vi "DataLog Format Stats.vi"(1 "tag config":T2 {"logging parameters" format="%.2e"; "precision" items=["0", "1", "2", "3", "4", "5", "6", "7", "8", "9", "10", "11", "12", "13", "14", "15", "16", "17"]; "limit delay" format="%.2e"; "deadband" format="%.2e"}, 2 "points":T1[](array[typedef]) {"value" format="%.3e"; "time" format="%<%H:%M:%S%2u\n%Y/%m/%d>T"}) -> (0 "stats":string)   [LabVIEW 2012]
doc: "Calculates statistics over a series of points. Formats the results to a display string."
uses:
  typedefs/clusters/t_DataLog Tag Config.ctl
  typedefs/t_DataLog Temporal Types.ctl
  typedefs/t_DataLog Value Types.ctl
  typedefs/t_DataLog Numerical Format.ctl
  typedefs/t_DataLog Logging Algorithms.ctl
  typedefs/clusters/t_DataLog Point.ctl
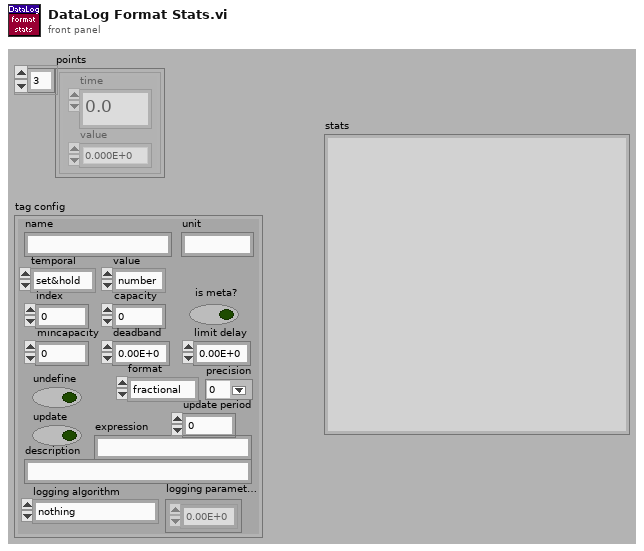
[diagram p1: front panel]
types:
  T1 = typedef "t_DataLog Point.ctl" = cluster{"time":dbl, "value":dbl}
  T2 = typedef "t_DataLog Tag Config.ctl" = cluster{"name":string, "unit":string, "temporal":T3, "value":T4, "index":i32, "capacity":i32, "is meta?":bool, "mincapacity":i32, "deadband":dbl, "limit delay":dbl, "format":T5, "precision":u8, "undefine":bool, "update":bool, "update period":u16, "expression":string, "description":string, "logging algorithm":T6, "logging parameters":dbl[]}
  T3 = typedef "t_DataLog Temporal Types.ctl" = enum16{"set&hold", "sample", "event"}
  T4 = typedef "t_DataLog Value Types.ctl" = enum16{"number", "string"}
  T5 = typedef "t_DataLog Numerical Format.ctl" = enum8{"fractional", "exponential", "engineering"}
  T6 = typedef "t_DataLog Logging Algorithms.ctl" = enum16{"nothing", "changes", "everything", "every Nth", "time threshold", "value threshold + prior", "t or v threshold", "t or v threshold + prior"}
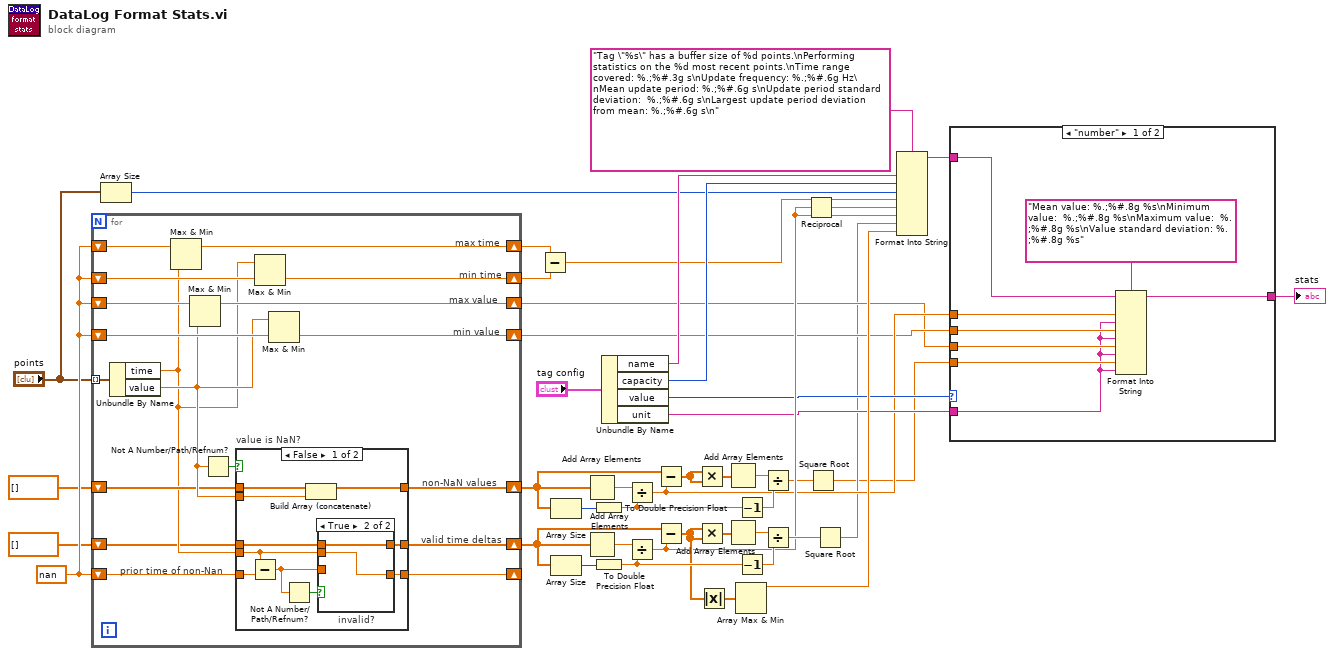
[diagram p0: block diagram]
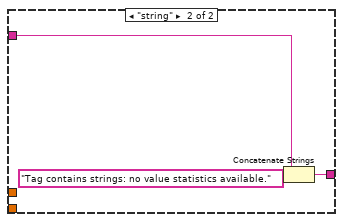
[diagram p2: hidden frame]
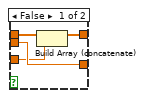
[diagram p3: hidden frame]
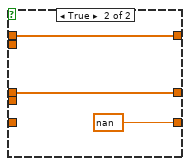
[diagram p4: hidden frame]
diagram:
  w43 = nan ("time")
  n1 = for {
    tunnel: "points" -> [w61] mode=indexing
    shift-right: [w55] -> w4
    shift-left: w43 -> [w56]
    shift-right: [w54] -> w5
    shift-left: w43 -> [w53]
    shift-right: [w59] -> w22
    shift-left: w43 -> [w60]
    shift-right: [w57] -> w21
    shift-left: w43 -> [w58]
    shift-right: [w51] -> w33
    shift-left: dbl[] [] -> [w49]
    shift-right: [w48] -> _
    shift-left: w43 -> [w47]
    shift-right: [w44] -> w31
    shift-left: dbl[] [] -> [w45]
    # "valid time deltas"
    # "prior time of non-Nan"
    # "non-NaN values"
    # "min value"
    # "max value"
    # "min time"
    # "max time"
    n2 = Unbundle By Name(w61) -> ("time"=w46:dbl, "value"=w50:dbl)
    n3 = Max & Min(x=w60, y=w46) -> (max(x,y)=w59:dbl)  [unwired: 1 out]
    n4 = Max & Min(x=w56, y=w50) -> (max(x,y)=w55:dbl)  [unwired: 1 out]
    n5 = Not A Number/Path/Refnum?(number/path/refnum=w50) -> (NaN/Path/Refnum?=w52:bool)
    n6 = case "value is NaN?" shown="False" w52 {
      tunnel: [w71 w80] -> w51
      tunnel: w50 -> [w70 _]
      tunnel: w49 -> [w69 w80]
      tunnel: [w65 nan ("time")] -> w48
      tunnel: w47 -> [w66 _]
      tunnel: w46 -> [w64 _]
      tunnel: w45 -> [w68 w78]
      tunnel: [w67 w78] -> w44
      frame False {
        n7 = Subtract(x=w64, y=w66) -> (x-y=w62:dbl)
        n8 = Not A Number/Path/Refnum?(number/path/refnum=w62) -> (NaN/Path/Refnum?=w63:bool)
        n9 = Build Array (concatenate)(w69, w70) -> (w71:dbl[])
        n10 = case "invalid?" shown="True" w63 {
          tunnel: w68 -> [w75 w77]
          tunnel: [w74 w77] -> w67
          tunnel: [w73 w76] -> w65
          tunnel: w64 -> [w73 w76]
          tunnel: w62 -> [w72 _]
          frame False {
            n11 = Build Array (concatenate)(w75, w72) -> (w74:dbl[])
          }
          frame True {
          }
        }
      }
      frame True {
      }
    }
    n12 = Max & Min(x=w46, y=w58) -> (min(x,y)=w57:dbl)  [unwired: 1 out]
    n13 = Max & Min(x=w50, y=w53) -> (min(x,y)=w54:dbl)  [unwired: 1 out]
  }
  n14 = Array Size(array="points") -> (size(s)=w16:i32)
  n15 = Subtract(x=w22, y=w21) -> (x-y=w15:dbl)
  n16 = Array Size(array=w33) -> (size(s)=w39:i32)
  n17 = Array Size(array=w31) -> (size(s)=w36:i32)
  n18 = Add Array Elements(numeric array=w33) -> (sum=w38:dbl)
  n19 = Add Array Elements(numeric array=w31) -> (sum=w37:dbl)
  n20 = To Double Precision Float(number=w39) -> (double precision float=w29:dbl)
  n21 = To Double Precision Float(number=w36) -> (double precision float=w30:dbl)
  n22 = Unbundle By Name("tag config") -> ("name"=w18:string, "capacity"=w17:i32, "value"=w9:T4, "unit"=w7:string)
  n23 = Divide(x=w38, y=w29) -> (x/y=w6:dbl)
  n24 = Divide(x=w37, y=w30) -> (x/y=w11:dbl)
  n25 = Subtract(x=w33, y=w6) -> (x-y=w35:dbl[])
  n26 = Subtract(x=w31, y=w11) -> (x-y=w24:dbl[])
  n27 = Multiply(x=w35, y=w35) -> (x*y=w34:dbl[])
  n28 = Multiply(x=w24, y=w24) -> (x*y=w32:dbl[])
  n29 = Absolute Value(x=w24) -> (abs(x)=w23:dbl[])
  n30 = Add Array Elements(numeric array=w34) -> (sum=w26:dbl)
  n31 = Add Array Elements(numeric array=w32) -> (sum=w28:dbl)
  n32 = Array Max & Min(array=w23) -> (max value=w13:dbl)  [unwired: 3 out]
  n33 = Decrement(x=w29) -> (x-1=w25:dbl)
  n34 = Decrement(x=w30) -> (x-1=w27:dbl)
  n35 = Divide(x=w26, y=w25) -> (x/y=w3:dbl)
  n36 = Divide(x=w28, y=w27) -> (x/y=w14:dbl)
  n37 = Reciprocal(x=w11) -> (1/x=w12:dbl)
  n38 = Square Root(x=w3) -> (sqrt(x)=w1:dbl)
  n39 = Square Root(x=w14) -> (sqrt(x)=w2:dbl)
  n40 = Format Into String(format string="Tag \"%s\" has a buffer size of %d points.\nPerforming statistics on the %d most recent points.\nTime range covered: %.;%#.3g s\nUpdate frequency: %.;%#.6g Hz\nMean update period: %.;%#.6g s\nUpdate period standard deviation:  %.;%#.6g s\nLargest update period deviation from mean: %.;%#.6g s\n", w18, w17, w16, w15, w12, w11, w2, w13) -> (resulting string=w10:string)  [unwired: 2 in, 1 out]
  n41 = case shown="\"number\"" w9 {
    tunnel: w10 -> [w88 w91]
    tunnel: [w87 w89] -> w8
    tunnel: w7 -> [w81 _]
    tunnel: w6 -> [w85 _]
    tunnel: w5 -> [w84 _]
    tunnel: w4 -> [w83 _]
    tunnel: w1 -> [w82 _]
    frame "number" {
      n42 = Format Into String(format string="Mean value: %.;%#.8g %s\nMinimum value:  %.;%#.8g %s\nMaximum value:  %.;%#.8g %s\nValue standard deviation: %.;%#.8g %s", initial string=w88, w85, w81, w84, w81, w83, w81, w82, w81) -> (resulting string=w87:string)  [unwired: 1 in, 1 out]
    }
    frame "string" {
      n43 = Concatenate Strings(w91, "Tag contains strings: no value statistics available." ("string")) -> (w89:string)
    }
  }
  "stats" <- w8
